vi "AFG3352X.update_mass services and attribute data for 2nd channel.vi"(0 "i ref in":refnum<vi>, 1 "frequency":dbl=1000.0, 2 "amplitude":dbl=0.1, 3 "ms timeout (10000)":i32=10000, 4 "phase":dbl, 5 "error in (no error)":errorcluster, 6 "enableOutput":bool=TRUE, 7 "DCOffset":dbl, 8 "trigger":i16[](array[numeric]), 9 "valueStatus":T1=enum."on", 10 "waveformType":T2) -> (14 "i ref out":refnum<vi>, 17 "timed out":bool, 19 "error out":errorcluster)   [LabVIEW 2014, in "AFG3352X.lvlib"]
doc: "Sets all my published services and internal data. This can be used to set default values for all services."
uses:
  AFG3352X.lvlib
  CS_Core/CSApplicationBaseClasses/AFGBase/AFGBase.waveformType.ctl
  CSlibraries/UtilityLib/UtilityLib.valueStatus.ctl
  CS_Core/CSApplicationBaseClasses/AFGBase/AFGBase.serviceType.ctl
  CS_Core/CSApplicationBaseClasses/AFGBase/AFGBase.directionType.ctl
  CS_Core/CSApplicationBaseClasses/AFGBase/AFGBase.lvlib
  CSlibraries/UtilityLib/UtilityLib.lvlib
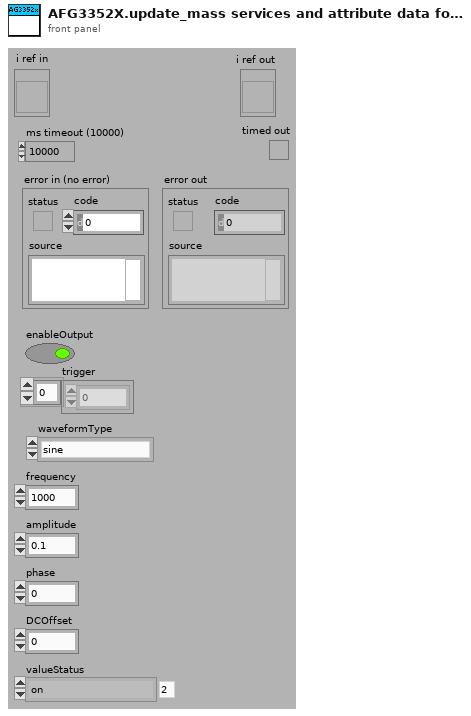
[diagram p1: front panel]
types:
  T1 = typedef "UtilityLib.lvlib/UtilityLib.valueStatus.ctl" = enum16{"no info available", "stand by/off", "on", "warning", "alarm/malfunction", "not implemented", "user action required", "important information", "system default", "control default", "indicator default", "button default"}
  T2 = typedef "AFGBase.lvlib/AFGBase.waveformType.ctl" = enum16{"sine", "square", "ramp", "pulse", "noise", "DC", "arbitrary", "triangle", "ramp_up", "ramp_down", "amplitude modulation"}
  T3 = typedef "AFGBase.lvlib/AFGBase.serviceType.ctl" = enum16{"frequency", "amplitude", "phase", "DCOffset", "enableOutput", "trigger", "waveformType"}
  T4 = typedef "AFGBase.lvlib/AFGBase.directionType.ctl" = enum16{"unknown", "update actual value", "update nominal value", "update both"}
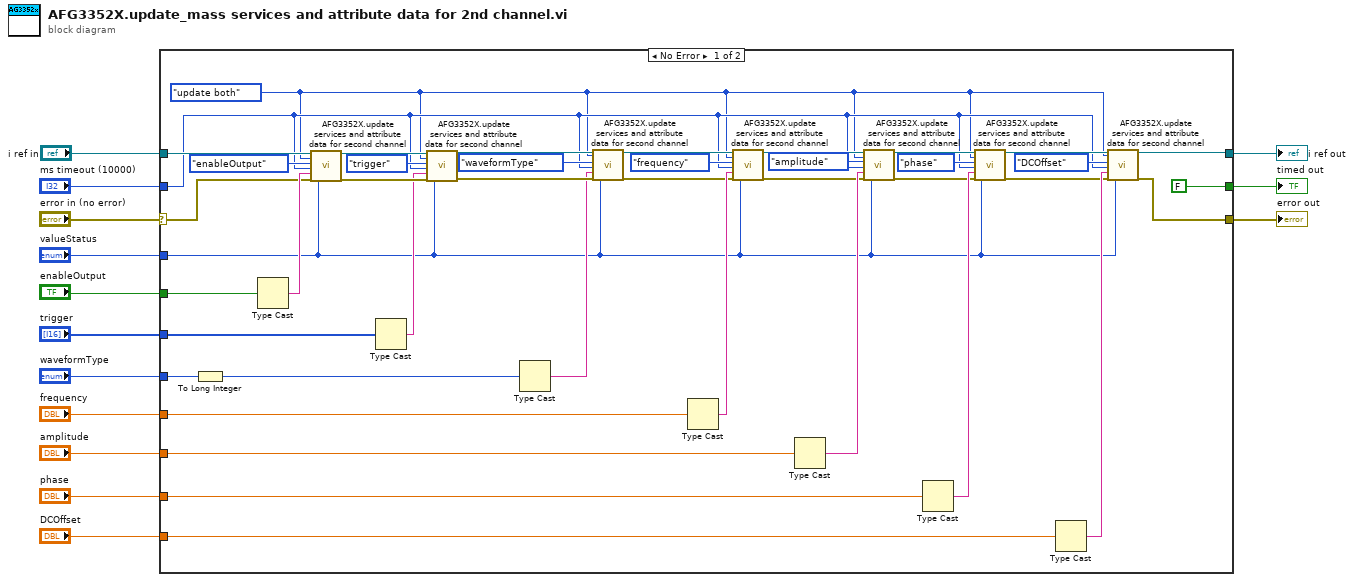
[diagram p0: block diagram]
diagram:
  n1 = case shown="No Error" "error in (no error)" {
    selector: "error in (no error)" -> [w48 w57]
    tunnel: [FALSE _] -> w14
    tunnel: [w28 w58] -> w1
    tunnel: "ms timeout (10000)" -> [w26 _]
    tunnel: "i ref in" -> [w49 w58]
    tunnel: [w27 w57] -> w11
    tunnel: "enableOutput" -> [w25 _]
    tunnel: "trigger" -> [w24 _]
    tunnel: "waveformType" -> [w22 _]
    tunnel: "frequency" -> [w21 _]
    tunnel: "amplitude" -> [w20 _]
    tunnel: "phase" -> [w19 _]
    tunnel: "DCOffset" -> [w18 _]
    tunnel: "valueStatus" -> [w15 _]
    frame No Error {
      w16 = AFGBase.directionType."update both" ("direction")
      n2 = To Long Integer(number=w22) -> (32bit integer=w17:i32)
      n3 = Type Cast(x=w25) -> (*(type *) &x=w55:string)  [unwired: 1 in]
      n4 = call "AFG3352X.update services and attribute data for second channel.vi"("i ref in"=w49, "direction"=w16, "service"=AFGBase.serviceType."enableOutput", "ms timeout (10000)"=w26, "value"=w55, "error in (no error)"=w48, "quality"=w15) -> ("i ref out"=w54:refnum<vi>, "error out"=w53:errorcluster)  [unwired: 10 in, 1 out]
      n5 = Type Cast(x=w24) -> (*(type *) &x=w23:string)  [unwired: 1 in]
      n6 = call "AFG3352X.update services and attribute data for second channel.vi"("i ref in"=w54, "direction"=w16, "service"=AFGBase.serviceType."trigger", "ms timeout (10000)"=w26, "value"=w23, "error in (no error)"=w53, "quality"=w15) -> ("i ref out"=w52:refnum<vi>, "error out"=w51:errorcluster)  [unwired: 10 in, 1 out]
      n7 = Type Cast(x=w17) -> (*(type *) &x=w50:string)  [unwired: 1 in]
      n8 = call "AFG3352X.update services and attribute data for second channel.vi"("i ref in"=w52, "direction"=w16, "service"=AFGBase.serviceType."waveformType", "ms timeout (10000)"=w26, "value"=w50, "error in (no error)"=w51, "quality"=w15) -> ("i ref out"=w46:refnum<vi>, "error out"=w45:errorcluster)  [unwired: 10 in, 1 out]
      n9 = Type Cast(x=w21) -> (*(type *) &x=w47:string)  [unwired: 1 in]
      n10 = call "AFG3352X.update services and attribute data for second channel.vi"("i ref in"=w46, "direction"=w16, "service"=AFGBase.serviceType."frequency", "ms timeout (10000)"=w26, "value"=w47, "error in (no error)"=w45, "quality"=w15) -> ("i ref out"=w43:refnum<vi>, "error out"=w42:errorcluster)  [unwired: 10 in, 1 out]
      n11 = Type Cast(x=w20) -> (*(type *) &x=w44:string)  [unwired: 1 in]
      n12 = call "AFG3352X.update services and attribute data for second channel.vi"("i ref in"=w43, "direction"=w16, "service"=AFGBase.serviceType."amplitude", "ms timeout (10000)"=w26, "value"=w44, "error in (no error)"=w42, "quality"=w15) -> ("i ref out"=w40:refnum<vi>, "error out"=w39:errorcluster)  [unwired: 10 in, 1 out]
      n13 = Type Cast(x=w19) -> (*(type *) &x=w41:string)  [unwired: 1 in]
      n14 = call "AFG3352X.update services and attribute data for second channel.vi"("i ref in"=w40, "direction"=w16, "service"=AFGBase.serviceType."phase", "ms timeout (10000)"=w26, "value"=w41, "error in (no error)"=w39, "quality"=w15) -> ("i ref out"=w30:refnum<vi>, "error out"=w29:errorcluster)  [unwired: 10 in, 1 out]
      n15 = Type Cast(x=w18) -> (*(type *) &x=w32:string)  [unwired: 1 in]
      n16 = call "AFG3352X.update services and attribute data for second channel.vi"("i ref in"=w30, "direction"=w16, "service"=AFGBase.serviceType."DCOffset", "ms timeout (10000)"=w26, "value"=w32, "error in (no error)"=w29, "quality"=w15) -> ("i ref out"=w28:refnum<vi>, "error out"=w27:errorcluster)  [unwired: 10 in, 1 out]
    }
    frame Error {
    }
  }
  "error out" <- w11
  "timed out" <- w14
  "i ref out" <- w1
